vi "Explore to Local Folder.vi"(8 "error in":errorcluster) -> (0 "error out":errorcluster)   [LabVIEW 2017, in "_Try Beta Version of CSMF.lvlib"]
uses:
  _Try Beta Version of CSMF.lvlib
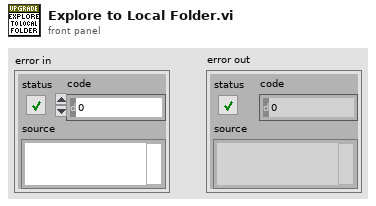
[diagram p1: front panel]
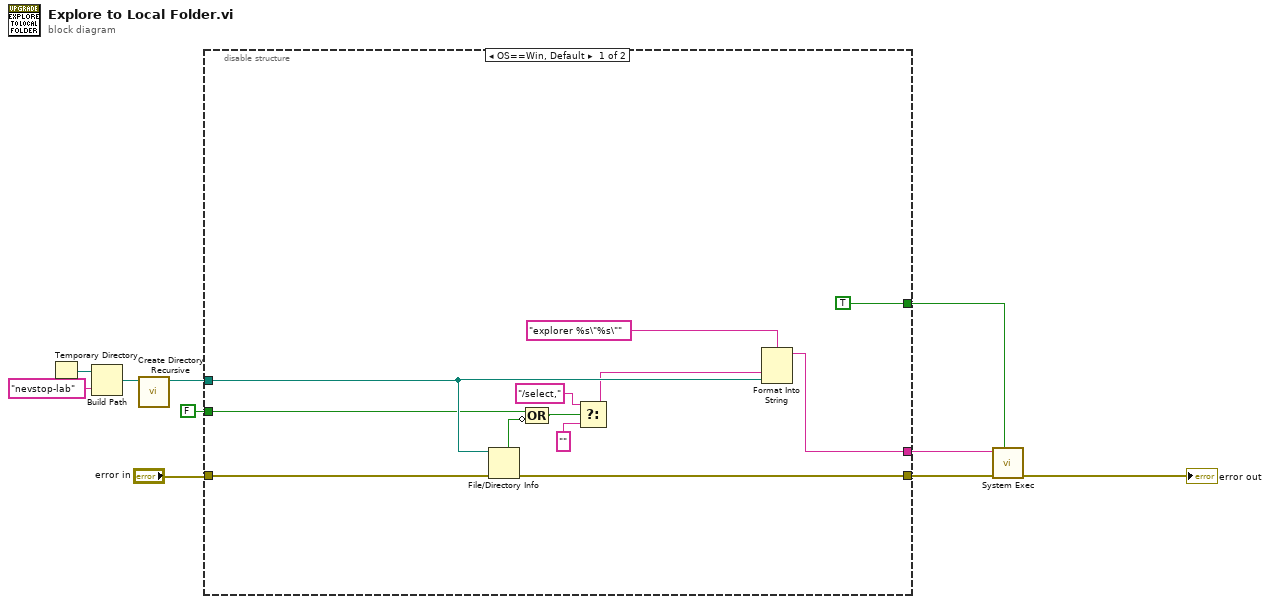
[diagram p0: block diagram]
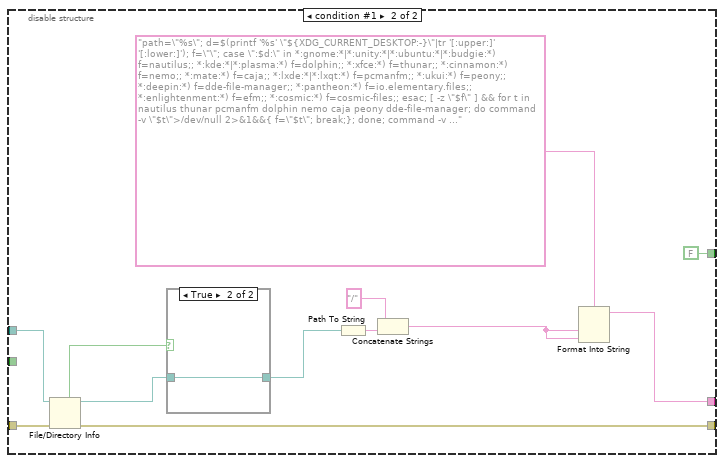
[diagram p2: hidden frame]
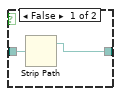
[diagram p3: hidden frame]
diagram:
  n1 = Temporary Directory() -> (w9:path)
  n2 = Build Path(base path=w9, name or relative path="nevstop-lab") -> (appended path=w8:path)
  n3 = call <vilib>:"Create Directory Recursive.vi"("directory"=w8) -> ("directory copy"=w5:path)  [unwired: 4 in, 2 out]
  n4 = disable-structure shown="OS==Win, Default" {
    disable-tunnel: w5 -> [w22 w26]
    disable-tunnel: [w17 w27] -> w4
    disable-tunnel: [w15 w33] -> w1
    disable-tunnel: "error in" -> [w13 w28]
    disable-tunnel: FALSE ("Select Directory? (F: Open Directory)") -> [w12 _]
    disable-tunnel: [TRUE ("wait until completion? (T)") FALSE ("wait until completion? (T)")] -> w2
    frame condition #0 (active) {
      n5 = File/Directory Info(path=w22, error in=w13) -> (directory=w16:bool, error out=w17:errorcluster)  [unwired: 5 out]
      n6 = Compound Arithmetic op=OR(w12, invert w16) -> (w18:bool)
      n7 = Select(t="/select," ("format string"), s=w18, f="") -> (s? t:f=w19:string)
      n8 = Format Into String(format string="explorer %s\"%s\"", w19, w22) -> (resulting string=w15:string)  [unwired: 2 in, 1 out]
    }
    frame condition #1 {
      n9 = File/Directory Info(path=w26, error in=w28) -> (path out=w25:path, directory=w24:bool, error out=w27:errorcluster)  [unwired: 4 out]
      n10 = case shown="True" w24 {
        tunnel: w25 -> [w36 w37]
        tunnel: [w35 w37] -> w23
        frame False {
          n11 = Strip Path(path=w36) -> (stripped path=w35:path)  [unwired: 1 out]
        }
        frame True {
        }
      }
      n12 = Path To String(path=w23) -> (string=w30:string)
      n13 = Concatenate Strings("/" ("string"), w30) -> (w29:string)
      n14 = Format Into String(format string="path=\"%s\"; d=$(printf '%s' \"${XDG_CURRENT_DESKTOP:-}\"|tr '[:upper:]' '[:lower:]'); f=\"\"; case \":$d:\" in *:gnome:*|*:unity:*|*:ubuntu:*|*:budgie:*) f=nautilus;; *:kde:*|*:plasma:*) f=dolphin;; *:xfce:*) f=thunar;; *:cinnamon:*) f=nemo;; *:mate:*) f=caja;; *:lxde:*|*:lxqt:*) f=pcmanfm;; *:ukui:*) f=peony;; *:deepin:*) f=dde-file-manager;; *:pantheon:*) f=io.elementary.files;; *:enlightenment:*) f=efm;; *:cosmic:*) f=cosmic-files;; esac; [ -z \"$f\" ] && for t in nautilus thunar pcmanfm dolphin nemo caja peony dde-file-manager; do command -v \"$t\">/dev/null 2>&1&&{ f=\"$t\"; break;}; done; command -v \"$f\">/dev/null 2>&1||f=xdg-open; [ \"$f\" = nautilus ] && nautilus --no-desktop \"$path\" 2>/dev/null||\"$f\" \"$path\"", w29, w29) -> (resulting string=w33:string)  [unwired: 2 in, 1 out]
    }
  }
  n15 = call <vilib>:"System Exec.vi"("wait until completion? (T)"=w2, "error in (no error)"=w4, "command line"=w1) -> ("error out"=→"error out":errorcluster)  [unwired: 5 in, 3 out]
